vi "TDO delay setting.vi"() -> ()   [LabVIEW 2017]
panel:
  in  "In":u8=1
  in  "error in (no error) 2":errorcluster
  in  "address":string="10.3.173.11"
  out "error out 2":errorcluster
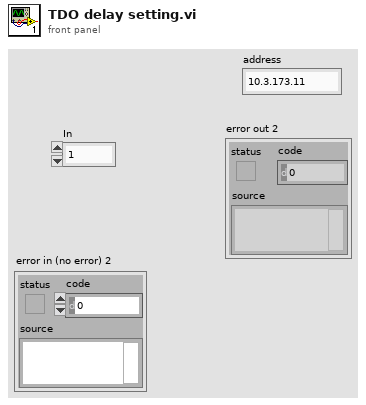
[diagram p1: front panel]
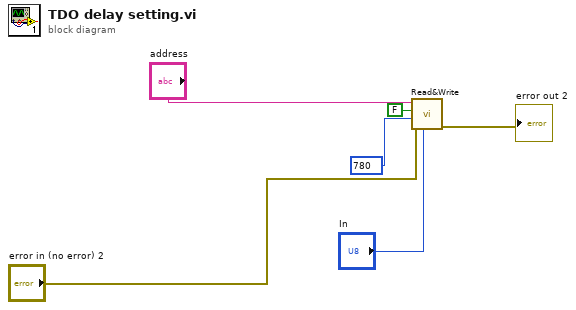
[diagram p0: block diagram]
diagram:
  n1 = call "Read&Write.vi"("In"="In", "error in (no error)"="error in (no error) 2", "Address"=u32 780, "Read (TRUE)"=FALSE, "address"="address") -> ("error out"=→"error out 2":errorcluster)  [unwired: 5 in, 1 out]
